vi "veristandSteps-lvDotNetConfigFile-update.vi"() -> ()   [LabVIEW 2014]
uses:
  <vilib>/xml/Load XML File.vi
  <vilib>/xml/Close Reference(Node).vi
  <vilib>/xml/Close Reference(NNMap).vi
  <vilib>/xml/NI_XML.lvlib
  <resource>/objmgr/DOMUserDefRef.rc
  <vilib>/ni/Simple XML/Simple XML.lvlib
  <vilib>/Wiresmith Technology/LabVIEW CLI/CLI Class/CLI.lvclass
panel:
  out "error out":errorcluster
  # "Arguments:\n1: Old EXE Config File\n2: New EXE Config File\n3: New TS Assembly Version\n4: New VS Assembly Version"
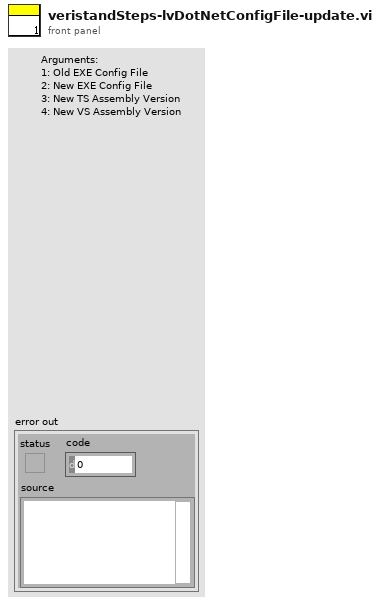
[diagram p1: front panel]
types:
  T1 = enum32{"invalid app kind", "Development System", "Run Time System", "Student Edition", "Embedded LabVIEW", "Evaluation", "Custom"}
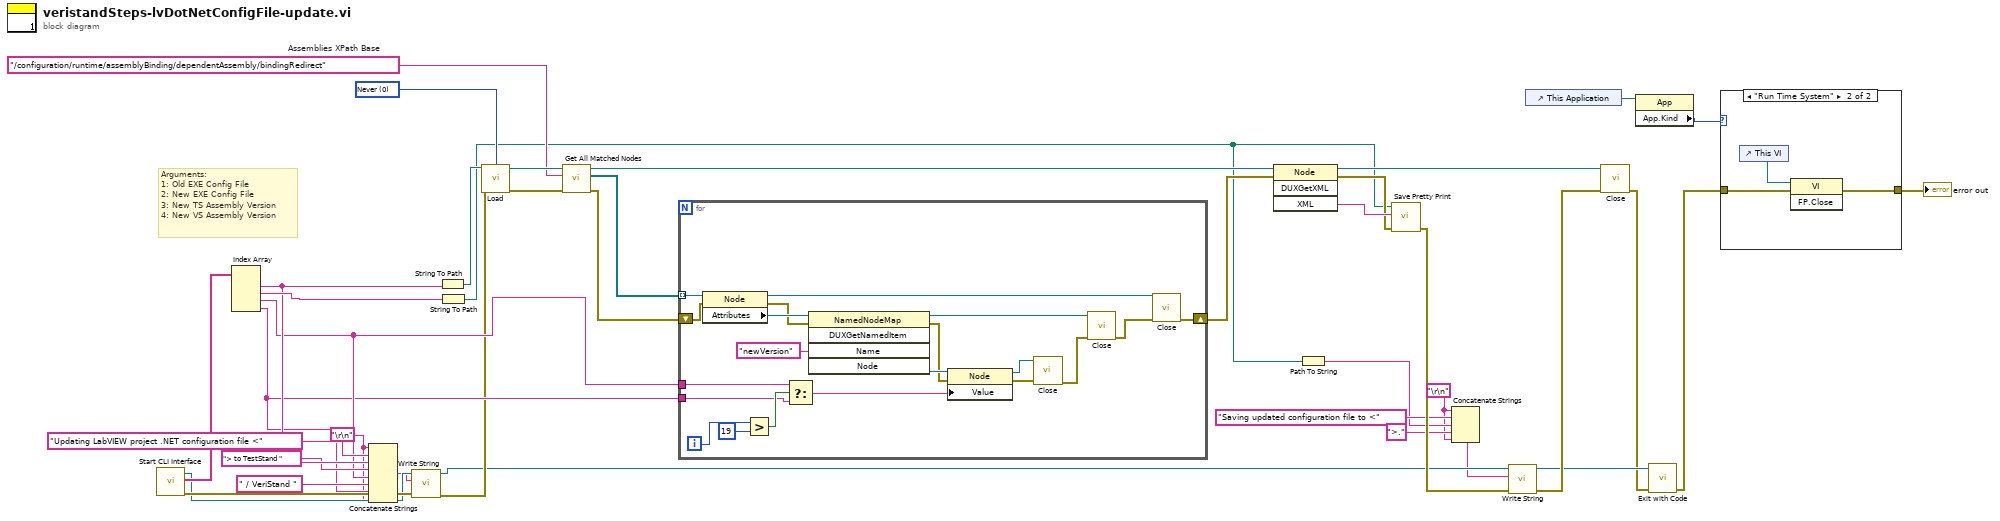
[diagram p0: block diagram]
diagram:
  w1 = "\r\n"
  w2 = "\r\n"
  w37 = "/configuration/runtime/assemblyBinding/dependentAssembly/bindingRedirect"  # Assemblies XPath Base
  w40 = 0 items=["Never", "Always", "Auto"] ("validate on load (Auto)")
  # "Arguments:\n1: Old EXE Config File\n2: New EXE Config File\n3: New TS Assembly Version\n4: New VS Assembly Version"
  n1 = call <vilib>:"Start CLI Interface.vi"() -> ("error out"=w23:errorcluster, "Custom Parameters"=w26:string[], "CLI out"=w15:refnum<class "CLI.lvclass">)  [unwired: 9 in]
  n2 = Index Array(array=w26) -> (element #1=w21:string, element #2=w25:string, element #3=w18:string, element #4=w17:string)  [unwired: 4 in]
  n3 = Concatenate Strings(w1, "Updating LabVIEW project .NET configuration file <", w21, "> to TestStand " ("string"), w18, " / VeriStand " ("string"), w17, w1) -> (w14:string)
  n4 = call <vilib>:"Write String.vi"("error in (no error)"=w23, "Text to Write"=w14, "CLI in"=w15) -> ("error out"=w16:errorcluster, "CLI out"=w12:refnum<class "CLI.lvclass">)  [unwired: 7 in]
  n5 = String To Path(string=w21) -> (path=w24:path)
  n6 = String To Path(string=w25) -> (path=w10:path)
  n7 = call-poly <vilib>:"Load.vi"("path to XML document"=w24, "validate on load (Auto)"=w40, "error in (no error)"=w16) -> ("DOM document out"=w38:refnum<k20>, "error out"=w39:errorcluster)  [unwired: 10 in, 1 out]
  n8 = call <vilib>:"Get All Matched Nodes.vi"("error in (no error)"=w39, "XPath expression"=w37, "node in"=w38) -> ("error out"=w35:errorcluster, "node result array"=w36:refnum<k20>[], "node out"=w33:refnum<k20>)  [unwired: 6 in]
  n9 = for {
    tunnel: w36 -> [w60] mode=indexing
    tunnel: w18 -> [w46]
    shift-right: [w48] -> w34
    shift-left: w35 -> [w57]
    tunnel: w17 -> [w41]
    i -> [w45]
    n10 = property class="Node"(reference=w60, error in=w57) -> (reference out=w50:refnum<k20>, error out=w58:errorcluster, "Attributes"=w59:refnum<k20>)
    n11 = Greater?(x=w45, y=19) -> (0:w43:bool)
    n12 = Select(t=w46, s=w43, f=w41) -> (s? t:f=w42:string)
    n13 = invoke class="NamedNodeMap" method="DUXGetNamedItem"(reference=w59, error in=w58, "Name"="newVersion") -> (reference out=w52:refnum<k20>, error out=w55:errorcluster, "Node"=w56:refnum<k20>)  [unwired: 2 in, 2 out]
    n14 = property class="Node"(reference=w56, error in=w55, "Value"=w42) -> (reference out=w53:refnum<k20>, error out=w54:errorcluster)
    n15 = call-poly <vilib>:"Close.vi"("error in (no error)"=w54, "node"=w53) -> ("error out"=w51:errorcluster)  [unwired: 7 in]
    n16 = call-poly <vilib>:"Close.vi"("error in (no error)"=w51, "named node map"=w52) -> ("error out"=w49:errorcluster)  [unwired: 7 in]
    n17 = call-poly <vilib>:"Close.vi"("error in (no error)"=w49, "node"=w50) -> ("error out"=w48:errorcluster)  [unwired: 7 in]
  }
  n18 = invoke class="Node" method="DUXGetXML"(reference=w33, error in=w34) -> (reference out=w30:refnum<k20>, error out=w31:errorcluster, "XML"=w32:string)  [unwired: 2 in, 1 out]
  n19 = Path To String(path=w10) -> (string=w9:string)
  n20 = call <vilib>:"Save Pretty Print.vi"("error in (no error)"=w31, "Pretty XML String"=w32, "XML file path"=w10) -> ("error out"=w13:errorcluster)  [unwired: 7 in, 1 out]
  n21 = Concatenate Strings(w2, "Saving updated configuration file to <" ("string"), w9, ">." ("string"), w2) -> (w7:string)
  n22 = call <vilib>:"Write String.vi"("error in (no error)"=w13, "Text to Write"=w7, "CLI in"=w12) -> ("error out"=w6:errorcluster, "CLI out"=w5:refnum<class "CLI.lvclass">)  [unwired: 7 in]
  n23 = control-ref of="This Application"() -> (w28:refnum<vi>)
  n24 = call-poly <vilib>:"Close.vi"("error in (no error)"=w6, "node"=w30) -> ("error out"=w4:errorcluster)  [unwired: 7 in]
  n25 = property class="App"(reference=w28) -> ("App.Kind"=w29:T1)  [unwired: 1 in, 2 out]
  n26 = call <vilib>:"Exit with Code.vi"("error in (no error)"=w4, "CLI in"=w5) -> ("error out"=w3:errorcluster)  [unwired: 9 in]
  n27 = case shown="\"Run Time System\"" w29 {
    tunnel: w3 -> [w61 w63]
    tunnel: [w61 w62] -> w27
    frame "Development System", Default {
    }
    frame "Run Time System" {
      n28 = control-ref of="This VI"() -> (w64:refnum<vi>)
      n29 = invoke class="VI" method="FP.Close"(reference=w64, error in=w63) -> (error out=w62:errorcluster)  [unwired: 1 in, 2 out]
    }
  }
  "error out" <- w27
